vi "Average.vi"(6 "Samples to average":i32=1, 10 "Data inn":T1={"Value"=nan, "Unit"="", "Status"=0} {"Value" format="%#.1f"}) -> (2 "Averaged data out":T1={"Value"=nan, "Unit"="", "Status"=0} {"Value" format="%#.1f"})   [LabVIEW 2011]
doc: "This VI averages data over a variable number of samples."
uses:
  Analog Var Disp 0 sif.ctl
  Status indicator Black Small.ctl
  <vilib>/Analysis/NI_AALBase.lvlib
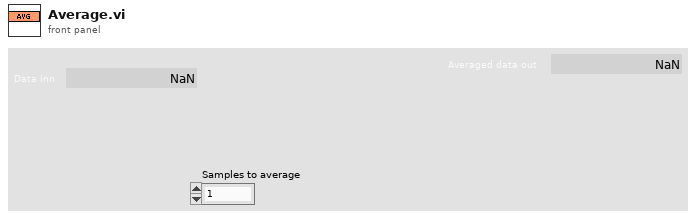
[diagram p1: front panel]
types:
  T1 = typedef "Analog Var Disp 0 sif.ctl" = cluster{"Value":dbl, "Unit":string, "Status":T2}
  T2 = typedef "Status indicator Black Small.ctl" = u16
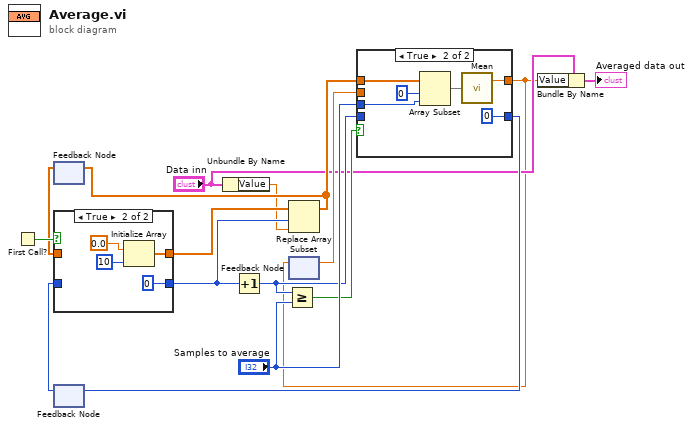
[diagram p0: block diagram]
diagram:
  n1 = First Call?() -> (First Call?: T/F=w15:bool)
  n2 = feedback #1() -> (w13:dbl[])  [unwired: 1 in]
  n3 = feedback #2() -> (w11:i32)  [unwired: 1 in]
  n4 = case shown="True" w15 {
    tunnel: [w17 w19] -> w14
    tunnel: w13 -> [w17 _]
    tunnel: [w16 0 ("index")] -> w12
    tunnel: w11 -> [w16 _]
    frame False {
    }
    frame True {
      n5 = Initialize Array(0.0 ("element"), 10 ("dimension size")) -> (w19:dbl[])
    }
  }
  n6 = Unbundle By Name("Data inn") -> ("Value"=w3:dbl)
  n7 = Increment(x=w12) -> (x+1=w6:i32)
  n8 = Greater Or Equal?(x=w6, y="Samples to average") -> (x >= y?=w8:bool)
  n9 = Replace Array Subset(array=w14, new element=w3, index=w12) -> (w10:dbl[])
  n10 = feedback-in #1(w10) -> ()
  n11 = feedback #3() -> (w5:dbl)  [unwired: 1 in]
  n12 = case shown="True" w8 {
    tunnel: w10 -> [_ w29]
    tunnel: "Samples to average" -> [_ w27]
    tunnel: [w23 0 ("t")] -> w7
    tunnel: w6 -> [w23 _]
    tunnel: [w22 w24] -> w2
    tunnel: w5 -> [w22 _]
    frame False {
    }
    frame True {
      n13 = Array Subset(array=w29, index=0, length=w27) -> (w26:dbl[])
      n14 = call <vilib>:"Mean.vi"("X"=w26) -> ("mean"=w24:dbl)  [unwired: 1 out]
    }
  }
  n15 = feedback-in #2(w7) -> ()
  n16 = feedback-in #3(w2) -> ()
  n17 = Bundle By Name(cluster="Data inn", "Value"=w2) -> (→"Averaged data out":T1)
